vi "Query Local Remote.vi"(7 "Slave Address":i32=-1 min=-1 max=30 step=1, 8 "error":errorcluster, 11 "VISA":refnum<visa-resource-name>) -> (0 "error out":errorcluster, 1 "Mode":enum32{"LOCAL", "REMOTE", "LOCKOUT"}(ring), 2 "Mode String":string, 3 "VISA out":refnum<visa-resource-name>)   [LabVIEW 2025, in "TDK-Lambda GEN LAN Series.lvlib"]
doc: "Reads the interface mode of the power supply. The response is given as an enumerated type and a string description. The mode string may be:\n\n(0) \"LOCAL\". The power-supply settings are made from its front panel buttons and knobs \n(1) \"REMOTE\". The power-supply settings are made using the LAN port. The \"Go to Local\" button may put the power supply into local mode\n(2) \"LOCKOUT\". Same as Remote but the \"Go to Local\" button will not operate\n\nIf a query error occured, Mode Str is set to be an empty string"
uses:
  <userlib>/TDK-Lambda GEN LAN Series/TDK-Lambda GEN LAN Series.lvlib
panel:
  # "TDK-Lambda Genesys \n LAN\n  DC Power Supplies"
  # "Read Mode:\n Local, Remote, or Lockout"
  # "(c) 2019 TDK-Lambda.  ALL RIGHTS RESERVED."
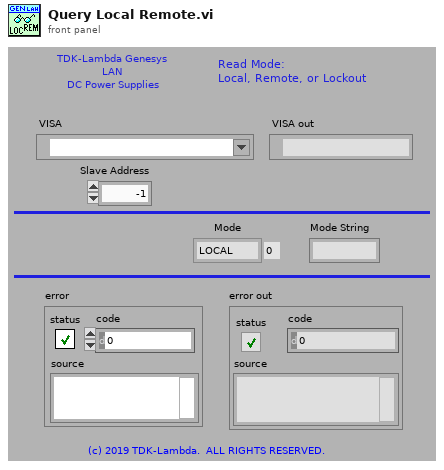
[diagram p1: front panel]
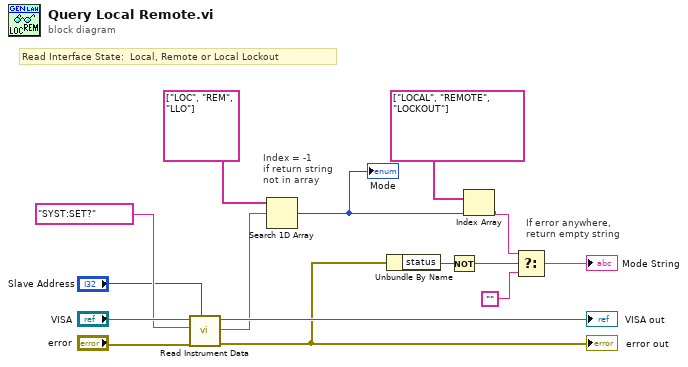
[diagram p0: block diagram]
diagram:
  # "If error anywhere,\nreturn empty string"
  # "Index = -1\nif return string\nnot in array"
  # "Read Interface State:  Local, Remote or Local Lockout"
  n1 = call <userlib>:"Read Instrument Data.vi"("Slave Address"="Slave Address", "error"="error", "Query"="SYST:SET?", "VISA"="VISA") -> ("error out"=w9:errorcluster, "Response"=w11:string, "VISA out"=→"VISA out":refnum<visa-resource-name>)  [unwired: 4 in, 1 out]
  "error out" <- w9
  n2 = Search 1D Array(1D array=string[] ["LOC", "REM", "LLO"], element=w11) -> (index of element=w2:i32)  [unwired: 1 in]
  "Mode" <- w2
  n3 = Unbundle By Name(w9) -> ("status"=w7:bool)
  n4 = Not(x=w7) -> (.not. x?=w8:bool)
  n5 = Index Array(array=string[] ["LOCAL", "REMOTE", "LOCKOUT"], index=w2) -> (element=w5:string)
  n6 = Select(t=w5, s=w8, f="") -> (s? t:f=→"Mode String":string)
